vi "数据插入.vi"(5 "数据类型":string(combo)="N", 7 "测量模式":string(combo), 8 "error in (no error)":errorcluster caption="错误输入（无错误）", 10 "data in":T1={"水样数据时间"=timestamp(0 s since 1904-01-01), "水样实测值"=0.0, "单位"="", "水样数据标识"="N", "信号值"=0.0, "标样参考值"=0.0, "因子编码"="", "探头温度"=0.0}, 11 "table输入":string(combo)) -> (0 "error out":errorcluster caption="错误输出")   [LabVIEW 2016, in "斯坦道多参数.lvlib"]
uses:
  <vilib>/Utility/sysdir.llb/System Directory Type.ctl
  <vilib>/Utility/error.llb/DialogType.ctl
  <vilib>/addons/database/Auxilliary.llb/DB Tools Transaction.ctl
  <vilib>/addons/database/Auxilliary.llb/DB Tools Isolation Level.ctl
  <vilib>/addons/database/Auxilliary.llb/DB Tools Column Info.ctl
  <vilib>/addons/database/Auxilliary.llb/DB Tools DataTypes.ctl
  <vilib>/addons/database/Auxilliary.llb/DB Tools Parameter Info.ctl
  <vilib>/addons/database/Auxilliary.llb/DB Tools Parameter Dir.ctl
  <vilib>/addons/database/Auxilliary.llb/DB Tools Format Datetime String (Time Stamp).vi
  <vilib>/addons/database/Connection.llb/DB Tools Open Connec (String).vi
  <vilib>/addons/database/Connection.llb/Conn Execute.vi
  <vilib>/addons/database/Recordset.llb/Rec Destroy - Connection.vi
  <vilib>/addons/database/Connection.llb/Conn Transaction.vi
  <vilib>/addons/database/Command.llb/Cmd Set Parameter Value (C).vi
  <vilib>/addons/database/Command.llb/Cmd Execute.vi
  <vilib>/addons/database/Recordset.llb/Rec Destroy - Command.vi
  <vilib>/addons/database/Command.llb/Cmd Delete.vi
  <vilib>/addons/database/NI_Database_API.lvlib
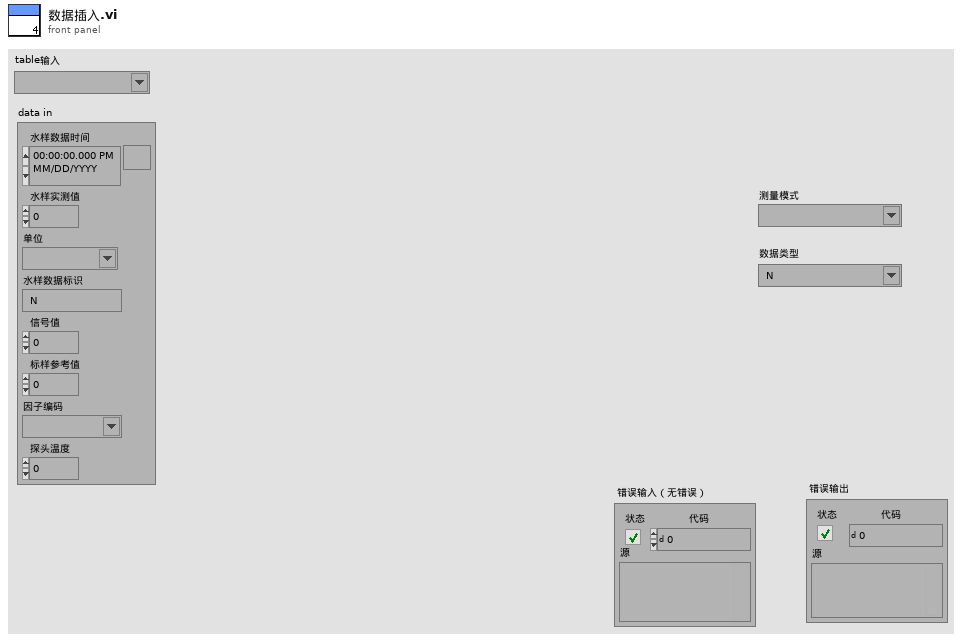
[diagram p1: front panel]
types:
  T1 = cluster{"水样数据时间":timestamp, "水样实测值":sgl, "单位":string, "水样数据标识":string, "信号值":sgl, "标样参考值":sgl, "因子编码":string, "探头温度":sgl}
  T2 = typedef "NI_Database_API.lvlib/DB Tools Parameter Info.ctl" = cluster{"parameter name":string, "type":T3, "direction":T4, "value":variant}
  T3 = typedef "NI_Database_API.lvlib/DB Tools DataTypes.ctl" = enum16{"String", "Long (I32)", "Single (SGL)", "Double (DBL)", "Date/Time", "Binary"}
  T4 = typedef "NI_Database_API.lvlib/DB Tools Parameter Dir.ctl" = enum32{"Input", "Output", "Input/Output", "Return Value"}
  T5 = typedef "NI_Database_API.lvlib/DB Tools Column Info.ctl" = cluster{"column name":string, "data type":T3, "size":i32, "allow null?":bool}
  T6 = typedef "NI_Database_API.lvlib/DB Tools Isolation Level.ctl" = enum16{"chaos", "read uncommitted", "read committed", "repeatable read", "serializable"}
  T7 = typedef "NI_Database_API.lvlib/DB Tools Transaction.ctl" = enum16{"begin", "commit", "rollback"}
  T8 = typedef "DialogType.ctl" = u16
  T9 = typedef "System Directory Type.ctl" = i32
  T10 = typedef "NI_Database_API.lvlib/Conn ObjectReference.ctl" = refnum<k1>
  T11 = typedef "NI_Database_API.lvlib/Rec ObjectReference.ctl" = refnum<k1>
  T12 = typedef "NI_Database_API.lvlib/Cmd ObjectReference.ctl" = refnum<k1>
  T13 = typedef "NI_Database_API.lvlib/Cmd-Rec Object Reference.ctl" = refnum<k1>
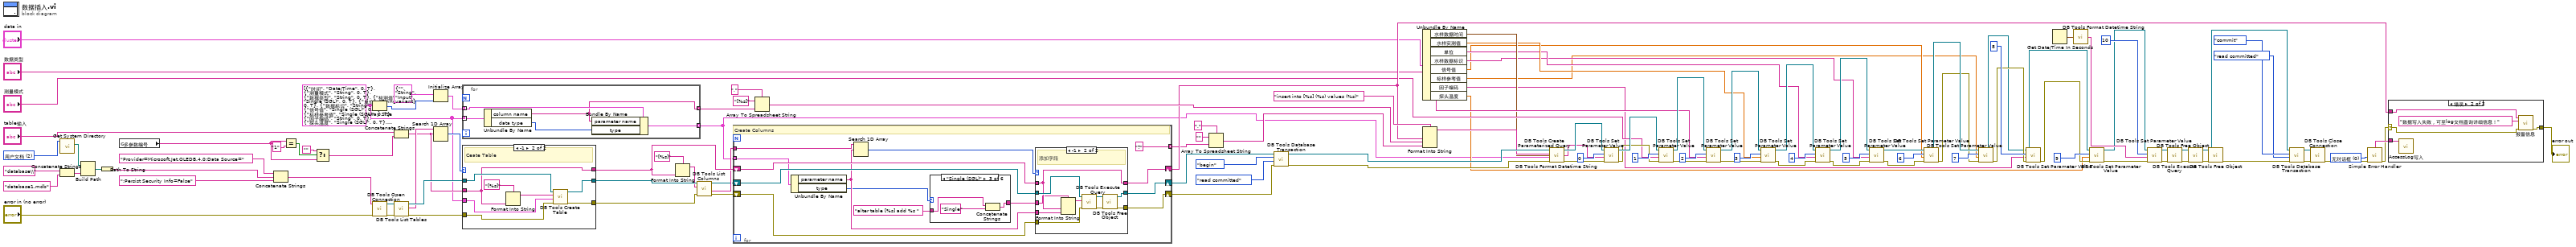
[diagram p0: block diagram]
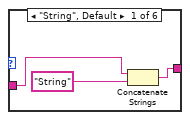
[diagram p2: hidden frame]
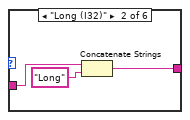
[diagram p3: hidden frame]
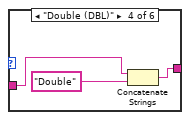
[diagram p4: hidden frame]
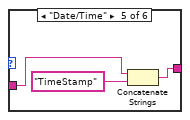
[diagram p5: hidden frame]
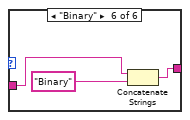
[diagram p6: hidden frame]
diagram:
  w1 = T5[] [{"column name"="时间", "data type"=enum."Date/Time", "size"=0, "allow null?"=TRUE}, {"column name"="测量模式", "data type"=enum."String", "size"=0, "allow null?"=TRUE}, {"column name"="数据类型", "data type"=enum."String", "size"=0, "allow null?"=TRUE}, {"column name"="检测值", "data type"=enum."Single (SGL)", "size"=0, "allow null?"=TRUE}, {"column name"="单位", "data type"=enum."String", "size"=0, "allow null?"=TRUE}, {"column name"="数据标识", "data type"=enum."String", "size"=0, "allow null?"=TRUE}, {"column name"="信号值", "data type"=enum."Single (SGL)", "size"=0, "allow null?"=TRUE}, {"column name"="标样参考值", "data type"=enum."Single (SGL)", "size"=0, "allow null?"=TRUE}, {"column name"="因子编码", "data type"=enum."String", "size"=0, "allow null?"=TRUE}, {"column name"="探头温度", "data type"=enum."Single (SGL)", "size"=0, "allow null?"=TRUE}, {"column name"="LastTime", "data type"=enum."Date/Time", "size"=0, "allow null?"=TRUE}] ("column information")
  w105 = T8 0 items=["无对话框", "确定信息", "继续或停止信息", "确定信息＋警告", "继续/停止+警告"] ("type of dialog (OK msg:1)")
  w118 = T9 2 items=["用户目录"=0, "用户桌面"=1, "用户文档"=2, "用户应用程序数据"=3, "用户设置"=4, "用户临时目录"=5, "公共文档"=6, "公共应用程序数据"=7, "公共设置"=8, "公共缓存"=13, "系统核心库"=9, "系统安装库"=10, "应用程序文件"=11, "启动盘根目录"=12] ("system directory type")
  n1 = call <vilib>:"Get System Directory.vi"("system directory type"=w118) -> ("system directory"=w116:path)  [unwired: 10 in]
  n2 = Concatenate Strings("database\\" ("condition"), "database1.mdb" ("字符串")) -> (w110:string)
  n3 = Build Path(base path=w116, name or relative path=w110) -> (appended path=w115:path)
  n4 = Path To String(path=w115) -> (string=w114:string)
  n5 = global read "多参数全局变量.vi" "多参数编号"() -> (w88:string)
  n6 = Concatenate Strings("Provider=Microsoft.Jet.OLEDB.4.0;Data Source=" ("condition"), w114, ";Persist Security Info=False" ("condition")) -> (w112:string)
  n7 = Equal?(x=w88, y="1") -> (x = y?=w90:bool)
  n8 = Select(t="", s=w90, f=w88) -> (s? t:f=w87:string)
  n9 = Array Size(array=w1) -> (size(s)=w5:i32)
  n10 = call-poly <vilib>:"DB Tools Open Connection.vi"("error in (no error)"="error in (no error)", "connection information"=w112) -> ("error out"=w97:errorcluster, "connection reference"=w108:T10)  [unwired: 6 in]
  n11 = Concatenate Strings("table输入", w87) -> (w80:string)
  n12 = call <vilib>:"DB Tools List Tables.vi"("error in (no error)"=w97, "connection reference"=w108) -> ("error out"=w100:errorcluster, "tables"=w99:string[], "connection reference out"=w101:T10)  [unwired: 3 in]
  n13 = Initialize Array(T2 {"parameter name"="", "type"=enum."String", "direction"=enum."Input", "value"=variant} ("parameter information"), w5) -> (w4:T2[])
  n14 = Search 1D Array(1D array=w99, element=w80) -> (index of element=w98:i32)  [unwired: 1 in]
  n15 = for {
    tunnel: w1 -> [w123] mode=indexing
    tunnel: w4 -> [w122] mode=indexing
    tunnel: [w120] -> w3 mode=indexing
    tunnel: [w119] -> w2 mode=indexing
    n16 = Unbundle By Name(w123) -> ("column name"=w119:string, "data type"=w121:T3)
    n17 = Bundle By Name(cluster=w122, "parameter name"=w119, "type"=w121) -> (w120:T2)
  }
  n18 = case shown="-1" w98 {
    tunnel: [w126 w133] -> w35
    tunnel: [w124 w131] -> w33
    tunnel: [w125 w129] -> w34
    tunnel: w101 -> [w126 w134]
    tunnel: w100 -> [w124 w132]
    tunnel: w80 -> [w125 w129]
    tunnel: w1 -> [_ w127]
    frame 0, Default {
    }
    frame -1 {
      # "Ceate Table"
      n19 = Format Into String(format string="[%s]" ("格式字符串"), w129) -> (resulting string=w130:string)  [unwired: 2 in, 1 out]
      n20 = call <vilib>:"DB Tools Create Table.vi"("error in (no error)"=w132, "column information"=w127, "table"=w130, "connection reference"=w134) -> ("error out"=w131:errorcluster, "connection reference out"=w133:T10)  [unwired: 4 in]
    }
  }
  n21 = Format Into String(format string="[%s]" ("格式字符串"), w34) -> (resulting string=w28:string)  [unwired: 2 in, 1 out]
  n22 = call <vilib>:"DB Tools List Columns.vi"("error in (no error)"=w33, "table"=w28, "connection reference"=w35) -> ("error out"=w27:errorcluster, "columns"=w26:string[], "connection reference out"=w25:T10)  [unwired: 1 in, 1 out]
  n23 = for {
    tunnel: w26 -> [w142]
    shift-right: [w147] -> w32
    shift-left: w34 -> [w148]
    shift-right: [w145] -> w30
    shift-left: w27 -> [w143]
    shift-right: [w146] -> w31
    shift-left: w25 -> [w141]
    tunnel: ["?"] -> w7 mode=indexing
    tunnel: w3 -> [w139] mode=indexing
    # "Create Columns"
    n24 = Unbundle By Name(w139) -> ("parameter name"=w138:string, "type"=w137:T3)
    n25 = Search 1D Array(1D array=w142, element=w138) -> (index of element=w144:i32)  [unwired: 1 in]
    n26 = case shown="\"Single (SGL)\"" w137 {
      tunnel: "alter table [%s] add %s " -> [w151 w154 w157 w160 w163 w166]
      tunnel: [w150 w153 w156 w159 w162 w165] -> w135
      frame "String", Default {
        n27 = Concatenate Strings(w151, "String" ("字符串")) -> (w150:string)
      }
      frame "Long (I32)" {
        n28 = Concatenate Strings(w154, "Long" ("字符串")) -> (w153:string)
      }
      frame "Single (SGL)" {
        n29 = Concatenate Strings(w157, "Single" ("字符串")) -> (w156:string)
      }
      frame "Double (DBL)" {
        n30 = Concatenate Strings(w160, "Double" ("字符串")) -> (w159:string)
      }
      frame "Date/Time" {
        n31 = Concatenate Strings(w163, "TimeStamp" ("字符串")) -> (w162:string)
      }
      frame "Binary" {
        n32 = Concatenate Strings(w166, "Binary" ("字符串")) -> (w165:string)
      }
    }
    n33 = case shown="-1" w144 {
      tunnel: w141 -> [w169 w177]
      tunnel: w143 -> [w168 w176]
      tunnel: w138 -> [_ w175]
      tunnel: [w169 w173] -> w146
      tunnel: [w168 w172] -> w145
      tunnel: w148 -> [w167 w171]
      tunnel: [w167 w171] -> w147
      tunnel: w135 -> [_ w170]
      frame 0, Default {
      }
      frame -1 {
        # "添加字段"
        n34 = Format Into String(format string=w170, w171, w175) -> (resulting string=w174:string)  [unwired: 2 in, 1 out]
        n35 = call-poly <vilib>:"DB Tools Execute Query.vi"("error in (no error)"=w176, "SQL query"=w174, "connection reference"=w177) -> ("error out"=w178:errorcluster, "recordset reference"=w179:T11)  [unwired: 5 in]
        n36 = call-poly <vilib>:"DB Tools Free Object.vi"("error in (no error)"=w178, "recordset reference"=w179) -> ("error out"=w172:errorcluster, "connection reference"=w173:T10)  [unwired: 8 in]
      }
    }
  }
  n37 = Array To Spreadsheet String(delimiter (Tab)="," ("分隔符(Tab)"), array=w2, 3:"[%s]" ("格式字符串")) -> (spreadsheet string=w81:string)
  n38 = Array To Spreadsheet String(delimiter (Tab)="," ("分隔符(Tab)"), array=w7, 3:"" ("格式字符串")) -> (spreadsheet string=w76:string)
  n39 = call-poly <vilib>:"DB Tools Database Transaction.vi"("error in (no error)"=w30, "isolation level (chaos)"=DB_Tools_Isolation_Level."read committed", "operation (begin)"=DB_Tools_Transaction."begin", "connection reference"=w31) -> ("error out"=w84:errorcluster, "connection reference out"=w85:T10)  [unwired: 2 in]
  n40 = Unbundle By Name("data in") -> ("水样数据时间"=w20:timestamp, "水样实测值"=w19:sgl, "单位"=w18:string, "水样数据标识"=w17:string, "信号值"=w16:sgl, "标样参考值"=w15:sgl, "因子编码"=w14:string, "探头温度"=w8:sgl)
  n41 = Format Into String(format string="insert into [%s] (%s) values (%s)" ("格式字符串"), w32, w81, w76) -> (resulting string=w75:string)  [unwired: 2 in, 1 out]
  n42 = call-poly <vilib>:"DB Tools Format Datetime String.vi"("time stamp"=w20) -> ("date/time string"=w71:string)
  n43 = call <vilib>:"DB Tools Create Parameterized Query.vi"("error in (no error)"=w84, "parameters"=w3, "SQL query"=w75, "connection reference"=w85) -> ("error out"=w73:errorcluster, "command reference"=w74:T12)  [unwired: 3 in, 1 out]
  n44 = call-poly <vilib>:"DB Tools Set Parameter Value.vi"("error in (no error)"=w73, "value"=w71, "parameter index"=0, "command reference"=w74) -> ("error out"=w60:errorcluster, "command reference out"=w69:T12)  [unwired: 4 in]
  n45 = call-poly <vilib>:"DB Tools Set Parameter Value.vi"("error in (no error)"=w60, "value"="测量模式", "parameter index"=1, "command reference"=w69) -> ("error out"=w61:errorcluster, "command reference out"=w62:T12)  [unwired: 4 in]
  n46 = call-poly <vilib>:"DB Tools Set Parameter Value.vi"("error in (no error)"=w61, "value"="数据类型", "parameter index"=2, "command reference"=w62) -> ("error out"=w59:errorcluster, "command reference out"=w58:T12)  [unwired: 4 in]
  n47 = call-poly <vilib>:"DB Tools Set Parameter Value.vi"("error in (no error)"=w59, "value"=w19, "parameter index"=3, "command reference"=w58) -> ("error out"=w56:errorcluster, "command reference out"=w57:T12)  [unwired: 4 in]
  n48 = call-poly <vilib>:"DB Tools Set Parameter Value.vi"("error in (no error)"=w56, "value"=w18, "parameter index"=4, "command reference"=w57) -> ("error out"=w54:errorcluster, "command reference out"=w55:T12)  [unwired: 4 in]
  n49 = call-poly <vilib>:"DB Tools Set Parameter Value.vi"("error in (no error)"=w54, "value"=w17, "parameter index"=5, "command reference"=w55) -> ("error out"=w51:errorcluster, "command reference out"=w53:T12)  [unwired: 4 in]
  n50 = call-poly <vilib>:"DB Tools Set Parameter Value.vi"("error in (no error)"=w51, "value"=w16, "parameter index"=6, "command reference"=w53) -> ("error out"=w50:errorcluster, "command reference out"=w52:T12)  [unwired: 4 in]
  n51 = call-poly <vilib>:"DB Tools Set Parameter Value.vi"("error in (no error)"=w50, "value"=w15, "parameter index"=7, "command reference"=w52) -> ("error out"=w47:errorcluster, "command reference out"=w46:T12)  [unwired: 4 in]
  n52 = call-poly <vilib>:"DB Tools Set Parameter Value.vi"("error in (no error)"=w47, "value"=w14, "parameter index"=8, "command reference"=w46) -> ("error out"=w10:errorcluster, "command reference out"=w12:T12)  [unwired: 4 in]
  n53 = Get Date/Time In Seconds() -> (seconds since 1Jan1904=w24:timestamp)
  n54 = call-poly <vilib>:"DB Tools Format Datetime String.vi"("time stamp"=w24) -> ("date/time string"=w45:string)
  n55 = call-poly <vilib>:"DB Tools Set Parameter Value.vi"("error in (no error)"=w10, "value"=w8, "parameter index"=9, "command reference"=w12) -> ("error out"=w9:errorcluster, "command reference out"=w11:T12)  [unwired: 4 in]
  n56 = call-poly <vilib>:"DB Tools Set Parameter Value.vi"("error in (no error)"=w9, "value"=w45, "parameter index"=10, "command reference"=w11) -> ("error out"=w44:errorcluster, "command reference out"=w43:T12)  [unwired: 4 in]
  n57 = call-poly <vilib>:"DB Tools Execute Query.vi"("error in (no error)"=w44, "command reference"=w43) -> ("error out"=w41:errorcluster, "command-recordset reference"=w42:T13)  [unwired: 6 in]
  n58 = call-poly <vilib>:"DB Tools Free Object.vi"("error in (no error)"=w41, "command-recordset reference"=w42) -> ("error out"=w37:errorcluster, "command reference"=w40:T12)  [unwired: 8 in]
  n59 = call-poly <vilib>:"DB Tools Free Object.vi"("error in (no error)"=w37, "command reference"=w40) -> ("error out"=w36:errorcluster, "connection reference"=w39:T10)  [unwired: 8 in]
  n60 = call-poly <vilib>:"DB Tools Database Transaction.vi"("error in (no error)"=w36, "isolation level (chaos)"=DB_Tools_Isolation_Level."read committed", "operation (begin)"=DB_Tools_Transaction."commit", "connection reference"=w39) -> ("error out"=w94:errorcluster, "connection reference out"=w38:T10)  [unwired: 2 in]
  n61 = call <vilib>:"DB Tools Close Connection.vi"("error in (no error)"=w94, "connection reference"=w38) -> ("error out"=w106:errorcluster)  [unwired: 5 in]
  n62 = call <vilib>:"Simple Error Handler.vi"("type of dialog (OK msg:1)"=w105, "error in (no error)"=w106) -> ("error out"=w103:errorcluster, "message"=w104:string)  [unwired: 3 in, 3 out]
  n63 = case shown="错误" w103 {
    selector: w103 -> [w180 w181]
    tunnel: w104 -> [_ w183]
    tunnel: [w180 w185] -> w102
    tunnel: w32 -> [_ w184]
    frame No Error {
    }
    frame Error {
      n64 = call "AccessLog写入.vi"("Log"=w183) -> ()  [unwired: 11 in]
      n65 = call "报警信息.vi"("error in (no error)"=w181, "报警信息"="数据写入失败，可至log文档查询详细信息！", "设备"=w184) -> ("error out"=w185:errorcluster)  [unwired: 8 in]
    }
  }
  "error out" <- w102
